vi "IR_cam_subVI.vi"(11 "Bytes Read":u8[](array[numeric])) -> (3 "Numeric":dbl)   [LabVIEW 2021]
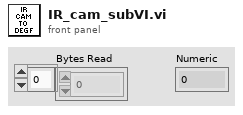
[diagram p1: front panel]
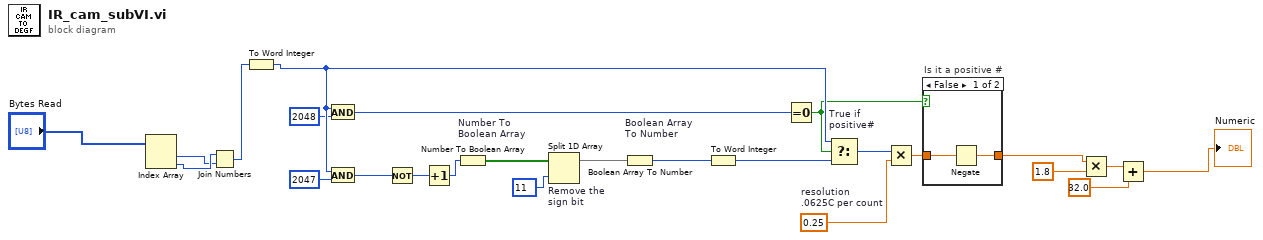
[diagram p0: block diagram]
diagram:
  w7 = 0.25  # resolution .0625C per count
  n1 = Index Array(array="Bytes Read") -> (element #1=w24:u8, element #2=w25:u8)  [unwired: 2 in]
  n2 = Join Numbers(hi=w25, lo=w24) -> ((hi.lo)=w23:u16)
  n3 = To Word Integer(number=w23) -> (16bit integer=w22:i16)
  n4 = And ("Out = 0x800\nif neg #")(x=w22, y=u16 2048 ("number 2")) -> (x .and. y?=w10:u16)
  n5 = And ("Just the \n12 bits")(x=w22, y=i16 2047 ("number")) -> (x .and. y?=w20:i16)
  n6 = Not(x=w20) -> (.not. x?=w11:i16)
  n7 = Increment(x=w11) -> (x+1=w12:i16)
  n8 = Number To Boolean Array "Number To\nBoolean Array"(number=w12) -> (Boolean array=w13:bool[])
  n9 = Split 1D Array "Remove the \nsign bit"(array=w13, index=11) -> (first subarray=w19:bool[])  [unwired: 1 out]
  n10 = Boolean Array To Number "Boolean Array \nTo Number"(Boolean array=w19) -> (number=w15:u32)
  n11 = To Word Integer(number=w15) -> (16bit integer=w16:i16)
  n12 = Equal To 0?(x=w10) -> (x = 0?=w17:bool)
  n13 = Select "True if \npositive#"(t=w22, s=w17, f=w16) -> (s? t:f=w9:i16)
  n14 = Multiply(x=w9, y=w7) -> (x*y=w18:dbl)
  n15 = case "Is it a positive #" shown="False" w17 {
    tunnel: w18 -> [w27 w28]
    tunnel: [w26 w28] -> w4
    frame False {
      n16 = Negate(x=w27) -> (-x=w26:dbl)
    }
    frame True {
    }
  }
  n17 = Multiply(x=w4, y=1.8) -> (x*y=w3:dbl)
  n18 = Add(x=w3, y=32.0) -> (x+y=→"Numeric":dbl)
